vi "HFRR ADV v01.vi"() -> ()   [LabVIEW 2025] (continued)
                      frame #16 {
                        n2627 = Wait (ms)(milliseconds to wait=u32 50) -> ()  [unwired: 1 out]
                      }
                      frame #17 {
                        n2628 = local read "USER ID"() -> (w3679:string)
                        n2629 = Concatenate Strings("Operator ID :" ("Content"), w3679) -> (w3681:string)
                        n2630 = local read "EVENT LOG"() -> (w3683:string)
                        n2631 = call "Event Log.vi"("Content"=w3681, "EVENT LOG"=w3683) -> ("EVENT LOG"=w3682:string)  [unwired: 8 in, 1 out]
                        n2632 = local write "EVENT LOG"(w3682) -> ()
                      }
                      frame #18 {
                        n2633 = Wait (ms)(milliseconds to wait=u32 50) -> ()  [unwired: 1 out]
                      }
                      frame #19 {
                        n2634 = disable-structure shown="Disabled" {
                          frame Disabled {
                            n2635 = local read "EVENT LOG"() -> (w3687:string)
                            n2636 = call "Event Log.vi"("Content"="Test Parameter", "EVENT LOG"=w3687) -> ("EVENT LOG"=w3686:string)  [unwired: 8 in, 1 out]
                            n2637 = local write "EVENT LOG"(w3686) -> ()
                          }
                          frame Enabled {
                          }
                        }
                      }
                      frame #20 {
                        n2638 = Wait (ms)(milliseconds to wait=u32 50) -> ()  [unwired: 1 out]
                      }
                      frame #21 {
                        n2639 = local read "Set Hz"() -> (w3691:dbl)
                        n2640 = Number To Fractional String(number=w3691, precision (6)=i16 2) -> (F-format string=w3690:string)  [unwired: 2 in]
                        n2641 = Concatenate Strings("Set Frequency [Hz] :" ("Content"), w3690) -> (w3693:string)
                        n2642 = local read "EVENT LOG"() -> (w3695:string)
                        n2643 = call "Event Log.vi"("Content"=w3693, "EVENT LOG"=w3695) -> ("EVENT LOG"=w3694:string)  [unwired: 8 in, 1 out]
                        n2644 = local write "EVENT LOG"(w3694) -> ()
                      }
                      frame #22 {
                        n2645 = Wait (ms)(milliseconds to wait=u32 50) -> ()  [unwired: 1 out]
                      }
                      frame #23 {
                        n2646 = local read "NORMAL LOAD"() -> (w3698:dbl)
                        n2647 = Number To Fractional String(number=w3698, precision (6)=i16 2) -> (F-format string=w3699:string)  [unwired: 2 in]
                        n2648 = Concatenate Strings("Applied Load [grams] :" ("Content"), w3699) -> (w3701:string)
                        n2649 = local read "EVENT LOG"() -> (w3703:string)
                        n2650 = call "Event Log.vi"("Content"=w3701, "EVENT LOG"=w3703) -> ("EVENT LOG"=w3702:string)  [unwired: 8 in, 1 out]
                        n2651 = local write "EVENT LOG"(w3702) -> ()
                      }
                      frame #24 {
                        n2652 = Wait (ms)(milliseconds to wait=u32 50) -> ()  [unwired: 1 out]
                      }
                      frame #25 {
                        n2653 = local read "Set Strk"() -> (w3706:dbl)
                        n2654 = Number To Fractional String(number=w3706, precision (6)=i16 2) -> (F-format string=w3707:string)  [unwired: 2 in]
                        n2655 = Concatenate Strings("Set Stroke [mm] :" ("Content"), w3707) -> (w3709:string)
                        n2656 = local read "EVENT LOG"() -> (w3711:string)
                        n2657 = call "Event Log.vi"("Content"=w3709, "EVENT LOG"=w3711) -> ("EVENT LOG"=w3710:string)  [unwired: 8 in, 1 out]
                        n2658 = local write "EVENT LOG"(w3710) -> ()
                      }
                      frame #26 {
                        n2659 = Wait (ms)(milliseconds to wait=u32 50) -> ()  [unwired: 1 out]
                      }
                      frame #27 {
                        n2660 = local read "Set Temp"() -> (w3714:dbl)
                        n2661 = Number To Fractional String(number=w3714, precision (6)=i16 2) -> (F-format string=w3715:string)  [unwired: 2 in]
                        n2662 = Concatenate Strings("Set Temperature [deg C] :" ("Content"), w3715) -> (w3717:string)
                        n2663 = local read "EVENT LOG"() -> (w3719:string)
                        n2664 = call "Event Log.vi"("Content"=w3717, "EVENT LOG"=w3719) -> ("EVENT LOG"=w3718:string)  [unwired: 8 in, 1 out]
                        n2665 = local write "EVENT LOG"(w3718) -> ()
                      }
                      frame #28 {
                        n2666 = Wait (ms)(milliseconds to wait=u32 50) -> ()  [unwired: 1 out]
                      }
                      frame #29 {
                        n2667 = local read "Set Rh"() -> (w3722:dbl)
                        n2668 = Number To Fractional String(number=w3722, precision (6)=i16 2) -> (F-format string=w3723:string)  [unwired: 2 in]
                        n2669 = Concatenate Strings("Set Humidity [%RH] :" ("Content"), w3723) -> (w3725:string)
                        n2670 = local read "EVENT LOG"() -> (w3727:string)
                        n2671 = call "Event Log.vi"("Content"=w3725, "EVENT LOG"=w3727) -> ("EVENT LOG"=w3726:string)  [unwired: 8 in, 1 out]
                        n2672 = local write "EVENT LOG"(w3726) -> ()
                      }
                      frame #30 {
                        n2673 = Wait (ms)(milliseconds to wait=u32 50) -> ()  [unwired: 1 out]
                      }
                      frame #31 {
                        n2674 = local read "test time"() -> (w3730:dbl)
                        n2675 = Number To Fractional String(number=w3730, precision (6)=i16 1) -> (F-format string=w3731:string)  [unwired: 2 in]
                        n2676 = Concatenate Strings("Test Duration [mins] :" ("Content"), w3731) -> (w3733:string)
                        n2677 = local read "EVENT LOG"() -> (w3735:string)
                        n2678 = call "Event Log.vi"("Content"=w3733, "EVENT LOG"=w3735) -> ("EVENT LOG"=w3734:string)  [unwired: 8 in, 1 out]
                        n2679 = local write "EVENT LOG"(w3734) -> ()
                      }
                      frame #32 {
                        w3736 = dbl[] [] ("History Data")
                        w3737 = cluster{"y":dbl, dbl, "y":dbl}[] [] ("History Data")
                        w3738 = FALSE ("Visible")
                        n2680 = property on="Stroke ( mm )" class="WFChart (strict)"("History Data"=w3737) -> ()  [unwired: 2 in, 2 out]
                        n2681 = property on="Temperature ( Deg C )" class="WFChart (strict)"("History Data"=w3736) -> ()  [unwired: 2 in, 2 out]
                        n2682 = property on="Electrical Contact Resistance ( % )" class="WFChart (strict)"("History Data"=w3736) -> ()  [unwired: 2 in, 2 out]
                        n2683 = property on="Coefficient of Friction" class="WFChart (strict)"("History Data"=w3736) -> ()  [unwired: 2 in, 2 out]
                        n2684 = property on="Frictional Force ( N )" class="WFChart (strict)"("History Data"=w3736) -> ()  [unwired: 2 in, 2 out]
                        n2685 = property on="Coefficient of Friction" class="WFChart (strict)"("History Data"=w3736) -> ()  [unwired: 2 in, 2 out]
                        n2686 = property on="Frictional Force ( N )" class="WFChart (strict)"("History Data"=w3736) -> ()  [unwired: 2 in, 2 out]
                        n2687 = property on="Electrical Contact Resistance ( % )" class="WFChart (strict)"("History Data"=w3736) -> ()  [unwired: 2 in, 2 out]
                        n2688 = property on="Stroke ( mm )" class="WFChart (strict)"("History Data"=w3737) -> ()  [unwired: 2 in, 2 out]
                        n2689 = property on="Temperature ( Deg C )" class="WFChart (strict)"("History Data"=w3736) -> ()  [unwired: 2 in, 2 out]
                        n2690 = property on="Service Password Log" class="Str"("Visible"=w3738) -> ()  [unwired: 2 in, 2 out]
                        n2691 = property on="Password 3" class="Clust (strict)"("Visible"=w3738) -> ()  [unwired: 2 in, 2 out]
                      }
                    }
                    n2692 = stacked-sequence {
                      frame #0 {
                        n2693 = local write "Main Dashboard Buttons"(T1."Dashboard" ("Main Dashboard Buttons")) -> ()
                        n2694 = local write "Main Tab"(T4."Acquire" ("Main Tab")) -> ()
                      }
                      frame #1 {
                        n2695 = local write "EVENT LOG"("" ("EVENT LOG")) -> ()
                      }
                      frame #2 {
                        n2696 = Wait (ms)(milliseconds to wait=u32 50) -> ()  [unwired: 1 out]
                      }
                      frame #3 {
                        n2697 = disable-structure shown="Disabled" {
                          frame Disabled {
                            n2698 = local read "EVENT LOG"() -> (w3745:string)
                            n2699 = call "Event Log.vi"("Content"="Test Details", "EVENT LOG"=w3745) -> ("EVENT LOG"=w3744:string)  [unwired: 8 in, 1 out]
                            n2700 = local write "EVENT LOG"(w3744) -> ()
                          }
                          frame Enabled {
                          }
                        }
                      }
                      frame #4 {
                        n2701 = Wait (ms)(milliseconds to wait=u32 50) -> ()  [unwired: 1 out]
                      }
                      frame #5 {
                        n2702 = local read "FILE"() -> (w3747:string)
                        n2703 = Concatenate Strings("File Name :" ("Content"), w3747) -> (w3748:string)
                        n2704 = local read "EVENT LOG"() -> (w3751:string)
                        n2705 = call "Event Log.vi"("Content"=w3748, "EVENT LOG"=w3751) -> ("EVENT LOG"=w3750:string)  [unwired: 8 in, 1 out]
                        n2706 = local write "EVENT LOG"(w3750) -> ()
                      }
                      frame #6 {
                        n2707 = Wait (ms)(milliseconds to wait=u32 50) -> ()  [unwired: 1 out]
                      }
                      frame #7 {
                        n2708 = local read "Batch Ref Num :"() -> (w3753:string)
                        n2709 = Concatenate Strings("Batch Ref No :" ("Content"), w3753) -> (w3754:string)
                        n2710 = local read "EVENT LOG"() -> (w3757:string)
                        n2711 = call "Event Log.vi"("Content"=w3754, "EVENT LOG"=w3757) -> ("EVENT LOG"=w3756:string)  [unwired: 8 in, 1 out]
                        n2712 = local write "EVENT LOG"(w3756) -> ()
                      }
                      frame #8 {
                        n2713 = Wait (ms)(milliseconds to wait=u32 50) -> ()  [unwired: 1 out]
                      }
                      frame #9 {
                        n2714 = local read "tested by"() -> (w3759:string)
                        n2715 = Concatenate Strings("Tested By :" ("Content"), w3759) -> (w3760:string)
                        n2716 = local read "EVENT LOG"() -> (w3763:string)
                        n2717 = call "Event Log.vi"("Content"=w3760, "EVENT LOG"=w3763) -> ("EVENT LOG"=w3762:string)  [unwired: 8 in, 1 out]
                        n2718 = local write "EVENT LOG"(w3762) -> ()
                      }
                      frame #10 {
                        n2719 = Wait (ms)(milliseconds to wait=u32 50) -> ()  [unwired: 1 out]
                      }
                      frame #11 {
                        n2720 = local read "TEST STANDARD"() -> (w3766:T5)
                        n2721 = case shown="\"ASTM D6079\", Default" w3766 {
                          tunnel: ["ASTM D6079" "ISO 12156" "CEC F-096-A-06" "Custom"] -> w3765
                          frame "ASTM D6079", Default {
                          }
                          frame "ISO 12156" {
                          }
                          frame "CEC F-096-A-06" {
                          }
                          frame "Custom" {
                          }
                        }
                        n2722 = Concatenate Strings("Test Standard :" ("Content"), w3765) -> (w3767:string)
                        n2723 = local read "EVENT LOG"() -> (w3770:string)
                        n2724 = call "Event Log.vi"("Content"=w3767, "EVENT LOG"=w3770) -> ("EVENT LOG"=w3769:string)  [unwired: 8 in, 1 out]
                        n2725 = local write "EVENT LOG"(w3769) -> ()
                      }
                      frame #12 {
                        n2726 = Wait (ms)(milliseconds to wait=u32 50) -> ()  [unwired: 1 out]
                      }
                      frame #13 {
                        n2727 = local read "Fuel Discription :"() -> (w3776:string)
                        n2728 = Concatenate Strings("Fuel Description :" ("Content"), w3776) -> (w3777:string)
                        n2729 = local read "EVENT LOG"() -> (w3780:string)
                        n2730 = call "Event Log.vi"("Content"=w3777, "EVENT LOG"=w3780) -> ("EVENT LOG"=w3779:string)  [unwired: 8 in, 1 out]
                        n2731 = local write "EVENT LOG"(w3779) -> ()
                      }
                      frame #14 {
                        n2732 = Wait (ms)(milliseconds to wait=u32 50) -> ()  [unwired: 1 out]
                      }
                      frame #15 {
                        n2733 = local read "Remarks :"() -> (w3782:string)
                        n2734 = Concatenate Strings("Remarks :" ("Content"), w3782) -> (w3783:string)
                        n2735 = local read "EVENT LOG"() -> (w3786:string)
                        n2736 = call "Event Log.vi"("Content"=w3783, "EVENT LOG"=w3786) -> ("EVENT LOG"=w3785:string)  [unwired: 8 in, 1 out]
                        n2737 = local write "EVENT LOG"(w3785) -> ()
                      }
                      frame #16 {
                        n2738 = Wait (ms)(milliseconds to wait=u32 50) -> ()  [unwired: 1 out]
                      }
                      frame #17 {
                        n2739 = local read "USER ID"() -> (w3788:string)
                        n2740 = Concatenate Strings("Operator ID :" ("Content"), w3788) -> (w3790:string)
                        n2741 = local read "EVENT LOG"() -> (w3792:string)
                        n2742 = call "Event Log.vi"("Content"=w3790, "EVENT LOG"=w3792) -> ("EVENT LOG"=w3791:string)  [unwired: 8 in, 1 out]
                        n2743 = local write "EVENT LOG"(w3791) -> ()
                      }
                      frame #18 {
                        n2744 = Wait (ms)(milliseconds to wait=u32 50) -> ()  [unwired: 1 out]
                      }
                      frame #19 {
                        n2745 = disable-structure shown="Disabled" {
                          frame Disabled {
                            n2746 = local read "EVENT LOG"() -> (w3796:string)
                            n2747 = call "Event Log.vi"("Content"="Test Parameter", "EVENT LOG"=w3796) -> ("EVENT LOG"=w3795:string)  [unwired: 8 in, 1 out]
                            n2748 = local write "EVENT LOG"(w3795) -> ()
                          }
                          frame Enabled {
                          }
                        }
                      }
                      frame #20 {
                        n2749 = Wait (ms)(milliseconds to wait=u32 50) -> ()  [unwired: 1 out]
                      }
                      frame #21 {
                        n2750 = local read "Set Hz"() -> (w3800:dbl)
                        n2751 = Number To Fractional String(number=w3800, precision (6)=i16 2) -> (F-format string=w3799:string)  [unwired: 2 in]
                        n2752 = Concatenate Strings("Set Frequency [Hz] :" ("Content"), w3799) -> (w3802:string)
                        n2753 = local read "EVENT LOG"() -> (w3804:string)
                        n2754 = call "Event Log.vi"("Content"=w3802, "EVENT LOG"=w3804) -> ("EVENT LOG"=w3803:string)  [unwired: 8 in, 1 out]
                        n2755 = local write "EVENT LOG"(w3803) -> ()
                      }
                      frame #22 {
                        n2756 = Wait (ms)(milliseconds to wait=u32 50) -> ()  [unwired: 1 out]
                      }
                      frame #23 {
                        n2757 = local read "NORMAL LOAD"() -> (w3807:dbl)
                        n2758 = Number To Fractional String(number=w3807, precision (6)=i16 2) -> (F-format string=w3808:string)  [unwired: 2 in]
                        n2759 = Concatenate Strings("Applied Load [grams] :" ("Content"), w3808) -> (w3810:string)
                        n2760 = local read "EVENT LOG"() -> (w3812:string)
                        n2761 = call "Event Log.vi"("Content"=w3810, "EVENT LOG"=w3812) -> ("EVENT LOG"=w3811:string)  [unwired: 8 in, 1 out]
                        n2762 = local write "EVENT LOG"(w3811) -> ()
                      }
                      frame #24 {
                        n2763 = Wait (ms)(milliseconds to wait=u32 50) -> ()  [unwired: 1 out]
                      }
                      frame #25 {
                        n2764 = local read "Set Strk"() -> (w3815:dbl)
                        n2765 = Number To Fractional String(number=w3815, precision (6)=i16 2) -> (F-format string=w3816:string)  [unwired: 2 in]
                        n2766 = Concatenate Strings("Set Stroke [mm] :" ("Content"), w3816) -> (w3818:string)
                        n2767 = local read "EVENT LOG"() -> (w3820:string)
                        n2768 = call "Event Log.vi"("Content"=w3818, "EVENT LOG"=w3820) -> ("EVENT LOG"=w3819:string)  [unwired: 8 in, 1 out]
                        n2769 = local write "EVENT LOG"(w3819) -> ()
                      }
                      frame #26 {
                        n2770 = Wait (ms)(milliseconds to wait=u32 50) -> ()  [unwired: 1 out]
                      }
                      frame #27 {
                        n2771 = local read "Set Temp"() -> (w3823:dbl)
                        n2772 = Number To Fractional String(number=w3823, precision (6)=i16 2) -> (F-format string=w3824:string)  [unwired: 2 in]
                        n2773 = Concatenate Strings("Set Temperature [deg C] :" ("Content"), w3824) -> (w3826:string)
                        n2774 = local read "EVENT LOG"() -> (w3828:string)
                        n2775 = call "Event Log.vi"("Content"=w3826, "EVENT LOG"=w3828) -> ("EVENT LOG"=w3827:string)  [unwired: 8 in, 1 out]
                        n2776 = local write "EVENT LOG"(w3827) -> ()
                      }
                      frame #28 {
                        n2777 = Wait (ms)(milliseconds to wait=u32 50) -> ()  [unwired: 1 out]
                      }
                      frame #29 {
                        n2778 = local read "Set Rh"() -> (w3831:dbl)
                        n2779 = Number To Fractional String(number=w3831, precision (6)=i16 2) -> (F-format string=w3832:string)  [unwired: 2 in]
                        n2780 = Concatenate Strings("Set Humidity [%RH] :" ("Content"), w3832) -> (w3834:string)
                        n2781 = local read "EVENT LOG"() -> (w3836:string)
                        n2782 = call "Event Log.vi"("Content"=w3834, "EVENT LOG"=w3836) -> ("EVENT LOG"=w3835:string)  [unwired: 8 in, 1 out]
                        n2783 = local write "EVENT LOG"(w3835) -> ()
                      }
                      frame #30 {
                        n2784 = Wait (ms)(milliseconds to wait=u32 50) -> ()  [unwired: 1 out]
                      }
                      frame #31 {
                        n2785 = local read "test time"() -> (w3839:dbl)
                        n2786 = Number To Fractional String(number=w3839, precision (6)=i16 1) -> (F-format string=w3840:string)  [unwired: 2 in]
                        n2787 = Concatenate Strings("Test Duration [mins] :" ("Content"), w3840) -> (w3842:string)
                        n2788 = local read "EVENT LOG"() -> (w3844:string)
                        n2789 = call "Event Log.vi"("Content"=w3842, "EVENT LOG"=w3844) -> ("EVENT LOG"=w3843:string)  [unwired: 8 in, 1 out]
                        n2790 = local write "EVENT LOG"(w3843) -> ()
                      }
                      frame #32 {
                        w3845 = dbl[] [] ("History Data")
                        w3846 = cluster{"y":dbl, dbl, "y":dbl}[] [] ("History Data")
                        w3847 = FALSE ("Visible")
                        n2791 = property on="Stroke ( mm )" class="WFChart (strict)"("History Data"=w3846) -> ()  [unwired: 2 in, 2 out]
                        n2792 = property on="Temperature ( Deg C )" class="WFChart (strict)"("History Data"=w3845) -> ()  [unwired: 2 in, 2 out]
                        n2793 = property on="Electrical Contact Resistance ( % )" class="WFChart (strict)"("History Data"=w3845) -> ()  [unwired: 2 in, 2 out]
                        n2794 = property on="Coefficient of Friction" class="WFChart (strict)"("History Data"=w3845) -> ()  [unwired: 2 in, 2 out]
                        n2795 = property on="Frictional Force ( N )" class="WFChart (strict)"("History Data"=w3845) -> ()  [unwired: 2 in, 2 out]
                        n2796 = property on="Coefficient of Friction" class="WFChart (strict)"("History Data"=w3845) -> ()  [unwired: 2 in, 2 out]
                        n2797 = property on="Frictional Force ( N )" class="WFChart (strict)"("History Data"=w3845) -> ()  [unwired: 2 in, 2 out]
                        n2798 = property on="Electrical Contact Resistance ( % )" class="WFChart (strict)"("History Data"=w3845) -> ()  [unwired: 2 in, 2 out]
                        n2799 = property on="Stroke ( mm )" class="WFChart (strict)"("History Data"=w3846) -> ()  [unwired: 2 in, 2 out]
                        n2800 = property on="Temperature ( Deg C )" class="WFChart (strict)"("History Data"=w3845) -> ()  [unwired: 2 in, 2 out]
                        n2801 = property on="Service Password Log" class="Str"("Visible"=w3847) -> ()  [unwired: 2 in, 2 out]
                        n2802 = property on="Password 3" class="Clust (strict)"("Visible"=w3847) -> ()  [unwired: 2 in, 2 out]
                      }
                    }
                    "TEST FILE NAM,E SAVED" <- TRUE ("TEST FILE NAM,E SAVED")
                  }
                }
              }
            }
          }
        }
        n2803 = case shown="Default" w3110 {
          tunnel: w3112 -> [_ w3215]
          frame Default {
            n2804 = property on="DEMO" class="Bool (strict)"() -> ("Value"=w3212:bool)  [unwired: 2 in, 2 out]
            n2805 = case shown="False" w3212 {
              frame False {
                w3214 = 0.0 ("output")
                n2806 = local write "PID-out"(w3214) -> ()
                n2807 = local write "Frequency ( Hz )"(w3214) -> ()
              }
              frame True {
              }
            }
            n2808 = local write "STROKE Initialize"(TRUE ("STROKE Initialize")) -> ()
          }
          frame "Acquire" {
            n2809 = stacked-sequence {
              frame #0 {
                n2810 = property on="DEMO" class="Bool (strict)"() -> ("Value"=w3217:bool)  [unwired: 2 in, 2 out]
                n2811 = case shown="False" w3217 {
                  frame False {
                    n2812 = local read "Auto Start Test"() -> (w3218:bool)
                    n2813 = case shown="True" w3218 {
                      tunnel: "RUN" -> [w3239 w3242]
                      tunnel: [w3239 w3241] -> w3219
                      frame False {
                      }
                      frame True {
                        n2814 = local read "Auto Start Temp"() -> (w3240:bool)
                        n2815 = Or(x=w3242, y=w3240) -> (x .or. y?=w3241:bool)
                      }
                    }
                    n2816 = local read "clk"() -> (w3238:dbl)
                    n2817 = local read "Save"() -> (w3234:bool)
                    n2818 = Equal?(x=w3238, y=0.0) -> (x = y?=w3235:bool)
                    n2819 = And(x=w3235, y=w3234) -> (x .and. y?=w3236:bool)
                    n2820 = Not(x="Engage") -> (.not. x?=w3225:bool)
                    n2821 = case shown="False" w3219 {
                      tunnel: [0.0 w3266] -> w3221
                      frame False {
                        (unwired) TRUE ("Visible")
                        n2822 = local read "Auto Start Test"() -> (w3246:bool)
                        n2823 = local write "Start Time"(TRUE ("Start Time")) -> ()
                        n2824 = property on="Stroke 2" class="DigNum (strict)"("Visible"=FALSE) -> ()  [unwired: 2 in, 2 out]
                        n2825 = case shown="False" w3246 {
                          frame False {
                            n2826 = property on="Heater Button" class="Bool (strict)"("DisabledEnum"=T20."Enabled" ("Disabled")) -> ()  [unwired: 2 in, 2 out]
                            n2827 = property on="Humidity" class="Bool (strict)"("DisabledEnum"=T20."Enabled" ("Disabled")) -> ()  [unwired: 2 in, 2 out]
                          }
                          frame True {
                          }
                        }
                        n2828 = case shown="False" "TestCompFlg" {
                          frame False {
                            n2829 = local read "StartFlg"() -> (w3254:bool)
                            n2830 = case shown="True" w3254 {
                              frame False {
                              }
                              frame True {
                                n2831 = stacked-sequence {
                                frame #0 {
                                n2832 = local read "EVENT LOG"() -> (w3258:string)
                                n2833 = call "Event Log.vi"("Content"="Test was interrupted", "EVENT LOG"=w3258) -> ("EVENT LOG"=w3259:string)  [unwired: 8 in, 1 out]
                                n2834 = local write "EVENT LOG"(w3259) -> ()
                                n2835 = property on="RUN" class="Bool (strict)"("Visible"=TRUE) -> ()  [unwired: 2 in, 2 out]
                                n2836 = property on="Auto Start Test" class="Bool (strict)"("Visible"=TRUE) -> ()  [unwired: 2 in, 2 out]
                                }
                                frame #1 {
                                w3262 = FALSE ("StartFlg")
                                n2837 = property on="Heater Button" class="Bool (strict)"("Val(Sgnl)"=FALSE ("Value (Signaling)")) -> ()  [unwired: 2 in, 2 out]
                                n2838 = local write "Heater Button"(w3262) -> ()
                                n2839 = local write "StartFlg"(w3262) -> ()
                                n2840 = local write "Humidity"(w3262) -> ()
                                n2841 = local write "Humidity 2"(TRUE ("Humidity")) -> ()
                                }
                                frame #2 {
                                n2842 = local write "Due Write"("VC;0" ("Command")) -> ()
                                }
                                frame #3 {
                                n2843 = Wait (ms)(milliseconds to wait=u32 1500) -> ()  [unwired: 1 out]
                                }
                                frame #4 {
                                n2844 = local write "Due Write"("HE;0" ("Command")) -> ()
                                }
                                }
                              }
                            }
                          }
                          frame True {
                          }
                        }
                        n2845 = local write "String 14"("Test will autostart once parameters reach the set value." ("String 14")) -> ()
                      }
                      frame True {
                        (unwired) FALSE ("Visible")
                        n2846 = property on="Stroke 2" class="DigNum (strict)"("Visible"=TRUE) -> ()  [unwired: 2 in, 2 out]
                        n2847 = property on="STOP 2" class="Bool (strict)"("Disabled"=u8 2) -> ()  [unwired: 2 in, 2 out]
                        n2848 = local write "String 14"(" Running....." ("String 14")) -> ()
                        n2849 = property on="Heater Button" class="Bool (strict)"("DisabledEnum"=T20."Disabled and Grayed Out" ("Disabled")) -> ()  [unwired: 2 in, 2 out]
                        n2850 = property on="Humidity" class="Bool (strict)"("DisabledEnum"=T20."Disabled and Grayed Out" ("Disabled")) -> ()  [unwired: 2 in, 2 out]
                        n2851 = case shown="True" "Start Time" {
                          selector: "Start Time" -> [_ w3285]
                          frame False {
                          }
                          frame True {
                            n2852 = Not(x=w3285) -> (.not. x?=w3284:bool)
                            n2853 = local write "Start Time"(w3284) -> ()
                            n2854 = local read "EVENT LOG"() -> (w3286:string)
                            n2855 = call "Event Log.vi"("Content"="Test in progress", "EVENT LOG"=w3286) -> ("EVENT LOG"=w3288:string)  [unwired: 8 in, 1 out]
                            n2856 = local write "EVENT LOG"(w3288) -> ()
                          }
                        }
                        n2857 = disable-structure shown="Enabled" {
                          disable-tunnel: [w3277 w3283] -> w3266
                          frame Disabled {
                            n2858 = local read "Set Hz"() -> (w3280:dbl)
                            n2859 = call <vilib>:"Uniform White Noise Waveform.vi"() -> ("signal out"=w3279:waveform(dbl))  [unwired: 10 in, 1 out]
                            n2860 = Random Number (0-1)() -> (number: 0 to 1=w3276:dbl)
                            n2861 = Add(x=w3280, y=w3279) -> (x+y=w3278:waveform(dbl))
                            n2862 = Multiply(x=ext 0.01 ("y"), y=w3276) -> (x*y=w3274:ext)
                            n2863 = Multiply(x=w3278, y=w3274) -> (x*y=w3277:waveform(ext))
                          }
                          frame Enabled {
                            n2864 = call-poly <vilib>:"Random Number (Range).vi"("lower bound (0)"=49.89, "upper bound (100)"=50.8) -> ("number"=w3283:dbl)  [unwired: 9 in]
                          }
                        }
                        "StartFlg" <- TRUE ("StartFlg")
                      }
                    }
                    n2865 = case shown="True" w3236 {
                      frame False {
                      }
                      frame True {
                        n2866 = local write "clk"(10.0 ("clk")) -> ()
                        n2867 = Get Date/Time In Seconds() -> (seconds since 1Jan1904=w3291:timestamp)
                        n2868 = To Double Precision Float(number=w3291) -> (double precision float=w3289:dbl)
                        n2869 = local write "acq timer"(w3289) -> ()
                        n2870 = local write "act save time"(w3289) -> ()
                      }
                    }
                    n2871 = call "Elapsed Time"("Time Target (s)"="Countdown", "Reset"=w3225) -> ("Elapsed Time (s)"=w3230:dbl, "Time has Elapsed"=w3228:bool)  [unwired: 10 in, 6 out]
                    "Countdown 2" <- w3230
                    n2872 = Subtract(x=w3230, y=2.0) -> (x-y=w3233:dbl)
                    n2873 = Less?(x=w3233, y="Countdown") -> (x < y?=w3231:bool)
                    n2874 = And(x=w3231, y=w3228) -> (x .and. y?=w3227:bool)
                    n2875 = case shown="True" w3227 {
                      frame False {
                      }
                      frame True {
                        (unwired) dbl[] [] ("History Data")
                        n2876 = local write "Engage"(FALSE ("Engage")) -> ()
                        n2877 = local write "RUN"(TRUE ("RUN")) -> ()
                        n2878 = local read "Humidity ( %RH )"() -> (→"Rh Before":dbl)
                      }
                    }
                    n2879 = local read "Test \nStatus"() -> (w3223:bool)
                    n2880 = Select(t=w3221, s=w3223, f=0.0) -> (s? t:f=w3222:dbl)
                    n2881 = local write "Frequency ( Hz )"(w3222) -> ()
                  }
                  frame True {
                  }
                }
              }
              frame #1 {
                # "HC;1/0\nST;VALUE"
                # "Elapsed time\ncof\nstroke\nAir temp\nTemp\nHumidity"
                # "acq timer\n\nact save time"
                # "convert to microseconds"
                n2882 = property on="DEMO" class="Bool (strict)"() -> ("Value"=w3292:bool)  [unwired: 2 in, 2 out]
                n2883 = case shown="True" w3292 {
                  tunnel: [w3310 FALSE] -> w3297
                  tunnel: [w3309 0.0] -> w3296
                  frame False {
                    w3317 = 1000000.0 ("x")
                    n2884 = local read "Rate"() -> (w3313:dbl)
                    n2885 = Divide(x=w3317, y=w3313) -> (x/y=w3318:dbl)
                    n2886 = Get Date/Time In Seconds() -> (seconds since 1Jan1904=w3320:timestamp)
                    n2887 = local read "Samplingtime 2"() -> (w3301:dbl)
                    n2888 = local read "act save time"() -> (w3315:dbl)
                    n2889 = Divide(x=w3318, y=w3317) -> (x/y=w3316:dbl)
                    n2890 = To Double Precision Float(number=w3320) -> (double precision float=w3309:dbl)
                    n2891 = Add(x=w3315, y=w3301) -> (x+y=w3314:dbl)
                    n2892 = local read "acq timer"() -> (w3319:dbl)
                    n2893 = local read "COUNT"() -> (w3302:i32)
                    n2894 = Greater Or Equal?(x=w3309, y=w3314) -> (x >= y?=w3300:bool)
                    n2895 = Multiply(x=w3316, y=w3302) -> (x*y=w3308:dbl)
                    n2896 = Subtract(x=w3309, y=w3319) -> (x-y=w3311:dbl)
                    n2897 = local read "Save"() -> (w3312:bool)
                    n2898 = Add(x=w3311, y=w3308) -> (x+y=w3298:dbl)
                    "Elapsed time 3" <- w3298
                    n2899 = And(x=w3300, y=w3312) -> (x .and. y?=w3310:bool)
                    n2900 = Divide(x=w3298, y=60.0) -> (x/y=w3306:dbl)
                    n2901 = local read "Test \nStatus"() -> (w3299:bool)
                    n2902 = local read "clk"() -> (w3303:dbl)
                    n2903 = Equal?(x=w3303, y=10.0) -> (x = y?=w3305:bool)
                    n2904 = case shown="True" w3299 {
                      tunnel: w3306 -> [_ w3329]
                      tunnel: w3311 -> [_ w3339]
                      tunnel: [0.0 w3335] -> _
                      tunnel: w3305 -> [_ w3334]
                      tunnel: [0.0 w3333] -> _
                      tunnel: w3298 -> [_ w3333]
                      tunnel: w3309 -> [w3322 _]
                      frame False {
                        n2905 = local write "acq timer"(w3322) -> ()
                        n2906 = local write "Test Duration Status"(0.0 ("Test Duration Status")) -> ()
                      }
                      frame True {
                        n2907 = local write "Elapsed time"(w3329) -> ()
                        n2908 = local read "Set Hz"() -> (w3336:dbl)
                        n2909 = local read "test time"() -> (w3328:dbl)
                        n2910 = Multiply(x=w3339, y=w3336) -> (x*y=w3338:dbl)
                        n2911 = Greater?(x=w3329, y=w3328) -> (0:w3337:bool)
                        n2912 = Subtract(x=w3328, y=w3329) -> (x-y=w3327:dbl)
                        n2913 = case shown="False" w3334 {
                          tunnel: w3338 -> [w3340 _]
                          tunnel: [w3340 1.0] -> w3335
                          frame False {
                            n2914 = local write "Cycles elapsed"(w3340) -> ()
                          }
                          frame True {
                          }
                        }
                        n2915 = Multiply(x=w3327, y=60.0) -> (x*y=w3326:dbl)
                        n2916 = local write "Time Remaining"(w3326) -> ()
                        n2917 = local write "Remaining Time"(w3326) -> ()
                        n2918 = case shown="True" w3337 {
                          frame False {
                          }
                          frame True {
                            n2919 = stacked-sequence {
                              frame #0 {
                                w3345 = T20."Enabled" ("Disabled")
                                w3344 = FALSE ("TEST FILE NAM,E SAVED")
                                w3346 = "" ("FILE")
                                w3347 = TRUE ("Visible")
                                n2920 = local write "Humidity"(FALSE ("Humidity")) -> ()
                                n2921 = local write "RUN"(FALSE ("OK Button 2")) -> ()
                                n2922 = local write "Heater Button"(FALSE ("Heater Button")) -> ()
                                n2923 = local write "Auto Start Test"(FALSE ("Auto Start Test")) -> ()
                                n2924 = local write "TestCompFlg"(TRUE ("StpFlg")) -> ()
                                n2925 = local read "Humidity ( %RH )"() -> (→"Rh After":dbl)
                                n2926 = property on="STOP 2" class="Bool (strict)"("Disabled"=u8 0) -> ()  [unwired: 2 in, 2 out]
                                n2927 = local read "EVENT LOG"() -> (w3352:string)
                                n2928 = call "Event Log.vi"("Content"="Test Completed", "EVENT LOG"=w3352) -> ("EVENT LOG"=w3351:string)  [unwired: 8 in, 1 out]
                                n2929 = property on="RUN" class="Bool (strict)"("Visible"=w3347) -> ()  [unwired: 2 in, 2 out]
                                n2930 = property on="Auto Start Test" class="Bool (strict)"("Visible"=w3347) -> ()  [unwired: 2 in, 2 out]
                                n2931 = local write "Batch Ref Num :"(w3346) -> ()
                                n2932 = local write "FILE"(w3346) -> ()
                                n2933 = local write "EVENT LOG"(w3351) -> ()
                                n2934 = local write "TEST FILE NAM,E SAVED"(w3344) -> ()
                                n2935 = local write "Fuel Discription :"(w3346) -> ()
                                n2936 = local write "START TEMP"(w3344) -> ()
                                n2937 = local write "Remarks :"(w3346) -> ()
                                n2938 = local write "Main Dashboard Buttons"(T1."Imaging" ("Main Dashboard Buttons")) -> ()
                                n2939 = local write "Main Tab"(T4."Adv Scar" ("Main Tab")) -> ()
                                n2940 = property on="FRICVALZ 2" class="Bool (strict)"("DisabledEnum"=w3345) -> ()  [unwired: 2 in, 2 out]
                                n2941 = property on="FRICVALZ 3" class="Bool (strict)"("DisabledEnum"=w3345) -> ()  [unwired: 2 in, 2 out]
                                n2942 = property on="FRICVALZ 4" class="Bool (strict)"("DisabledEnum"=w3345) -> ()  [unwired: 2 in, 2 out]
                              }
                              frame #1 {
                                n2943 = Wait (ms)(milliseconds to wait=u32 2000) -> ()  [unwired: 1 out]
                              }
                              frame #2 {
                                n2944 = local write "Due Write"("VC;0") -> ()
                              }
                              frame #3 {
                                n2945 = Wait (ms)(milliseconds to wait=u32 2000) -> ()  [unwired: 1 out]
                              }
                              frame #4 {
                                n2946 = local write "Due Write"("VC;0") -> ()
                              }
                              frame #5 {
                                n2947 = Wait (ms)(milliseconds to wait=u32 2000) -> ()  [unwired: 1 out]
                              }
                              frame #6 {
                                n2948 = local write "Due Write"("ST;0") -> ()
                              }
                              frame #7 {
                                n2949 = local write "measured_stroke"(0.0 ("measured_stroke")) -> ()
                                n2950 = Wait (ms)(milliseconds to wait=u32 1500) -> ()  [unwired: 1 out]
                              }
                              frame #8 {
                                n2951 = local write "Due Write"("HE;0") -> ()
                                n2952 = local write "Humidity 2"(TRUE ("Humidity")) -> ()
                              }
                            }
                          }
                        }
                        n2953 = Divide(x=w3329, y=w3328) -> (x/y=w3332:dbl)
                        n2954 = Multiply(x=w3332, y=100.0) -> (x*y=w3330:dbl)
                        n2955 = local write "Test Duration Status"(w3330) -> ()
                      }
                    }
                  }
                  frame True {
                  }
                }
                n2956 = local read "COUNT"() -> (w3294:i32)
                n2957 = Greater Or Equal?(x=w3294, y=250) -> (x >= y?=w3293:bool)
                n2958 = case shown="True" w3293 {
                  frame False {
                    n2959 = local read "COUNT"() -> (w3370:i32)
                    n2960 = Increment(x=w3370) -> (x+1=w3371:i32)
                    n2961 = local write "COUNT"(w3371) -> ()
                  }
                  frame True {
                    n2962 = local write "COUNT"(0 ("COUNT")) -> ()
                  }
                }
                n2963 = case shown="True" w3297 {
                  tunnel: w3296 -> [_ w3438]
                  tunnel: [FALSE ("Boolean 2") TRUE ("Boolean 2")] -> _
                  frame False {
                  }
                  frame True {
                    w3392 = ";" ("Substring")
                    # "Pid out/\nFreq response value"
                    n2964 = local write "act save time"(w3438) -> ()
                    n2965 = local read "FILE"() -> (w3386:string)
                    n2966 = call "file check.vi"("file name in"=w3386) -> ("error out"=w3389:errorcluster, "file name out"=w3384:string)  [unwired: 9 in]
                    n2967 = local read "LVDT STROKE"() -> (w3381:dbl)
                    n2968 = local read "Add up Stroke"() -> (w3379:dbl)
                    n2969 = call "FILE PATH CREATION.vi"("error in"=w3389, "FILE NAME :"=w3384) -> ("FILE OUT"=w3387:path)  [unwired: 8 in, 1 out]
                    n2970 = local read "STROKE Initialize"() -> (w3374:bool)
                    n2971 = Concatenate Strings(w3384, ".dgf" ("Substring")) -> (w3388:string)
                    n2972 = Subtract(x=w3381, y=w3379) -> (x-y=w3380:dbl)
                    n2973 = Absolute Value(x=w3380) -> (abs(x)=w3377:dbl)
                    n2974 = local read "FF 2"() -> (→"Frictional Force ( N )" →"Frictional Force ( N )":dbl)
                    n2975 = Build Path(base path=w3387, name or relative path=w3388) -> (appended path=w3383:path)
                    n2976 = flat-sequence {
                      tunnel: w3377 -> [w3443]
                      tunnel: [w3442] -> w3375
                      tunnel: w3374 -> [w3440]
                      tunnel: [w3445] -> w3376
                      tunnel: w3375 -> [w3445]
                      frame #0 {
                        n2977 = call <vilib>:"Mean PtByPt.vi"("x"=w3443, "sample length"="STROKE FILTER", "initialize"=w3440) -> ("mean"=w3442:dbl)  [unwired: 1 in, 1 out]
                      }
                      frame #1 {
                        "STROKE Initialize" <- FALSE ("STROKE Initialize")
                      }
                    }
                    n2978 = local read "COF 2"() -> (w3397:dbl)
                    "Coefficient of Friction" <- w3397
                    "COF 4" <- w3397
                    "Coefficient of Friction" <- w3397
                    n2979 = local read "TEMP"() -> (w3400:dbl)
                    "Temperature ( Deg C )" <- w3400
                    n2980 = local read "Humidity ( %RH )"() -> (w3399:dbl)
                    n2981 = local read "Frequency ( Hz )"() -> (w3406:dbl)
                    n2982 = local read "LVDT STROKE DISPLAY"() -> (w3378:dbl)
                    n2983 = local read "Elapsed time"() -> (w3431:dbl)
                    n2984 = local read "AIR TEMP"() -> (w3404:dbl)
                    n2985 = local read "PID-out"() -> (w3409:dbl)
                    n2986 = local write "Temperature ( Deg C )"(w3400) -> ()
                    n2987 = Number To Fractional String(number=w3378, width (-)=i16 9 ("precision (6)"), precision (6)=i16 6) -> (F-format string=w3424:string)  [unwired: 1 in]
                    n2988 = Number To Fractional String(number=w3404, width (-)=i16 9 ("precision (6)"), precision (6)=i16 3) -> (F-format string=w3423:string)  [unwired: 1 in]
                    n2989 = Number To Fractional String(number=w3400, width (-)=i16 9 ("precision (6)"), precision (6)=i16 3) -> (F-format string=w3420:string)  [unwired: 1 in]
                    n2990 = Number To Fractional String(number=w3399, width (-)=i16 9 ("precision (6)"), precision (6)=i16 3) -> (F-format string=w3417:string)  [unwired: 1 in]
                    n2991 = Number To Fractional String(number=0.0, width (-)=i16 9 ("precision (6)"), precision (6)=i16 3) -> (F-format string=w3414:string)  [unwired: 1 in]
                    n2992 = Number To Fractional String(number=w3409, width (-)=i16 9 ("precision (6)"), precision (6)=i16 3) -> (F-format string=w3410:string)  [unwired: 1 in]
                    n2993 = Number To Fractional String(number=w3406, width (-)=i16 9 ("precision (6)"), precision (6)=i16 3) -> (F-format string=w3405:string)  [unwired: 1 in]
                    n2994 = Number To Fractional String(number=w3397, width (-)=i16 9 ("precision (6)"), precision (6)=i16 6) -> (F-format string=w3432:string)  [unwired: 1 in]
                    n2995 = Number To Fractional String(number=w3431, width (-)=i16 14 ("precision (6)"), precision (6)=i16 3) -> (F-format string=w3433:string)  [unwired: 1 in]
                    n2996 = Bundle("y"=1.02, "LVDT STROKE DISPLAY"=w3378, "y"=0.98) -> (w3398:T31)  [unwired: 1 in]
                    n2997 = Number To Fractional String(number="Ambient Humidity :", width (-)=i16 9 ("precision (6)"), precision (6)=i16 6) -> (F-format string=w3390:string)  [unwired: 1 in]
                    n2998 = local read "RUN"() -> (w3396:bool)
                    n2999 = case shown="True" w3396 {
                      tunnel: w3398 -> [_ w3449]
                      tunnel: w3378 -> [_ w3448]
                      tunnel: w3378 -> [_ w3446]
                      tunnel: w3378 -> [_ w3447]
                      frame False {
                      }
                      frame True {
                        "Stroke ( mm )" <- w3449
                        "Stroke ( mm )" <- w3449
                        "Stroke 4" <- w3448
                        "Stroke 3" <- w3446
                        "Stroke 2" <- w3447
                        "measured_stroke" <- w3446
                      }
                    }
                    n3000 = Concatenate Strings(w3433, w3392, w3432, w3392, w3424, w3392, w3423, w3392, w3420, w3392, w3417, w3392, w3414, w3392, w3410, w3392, w3405, w3392, w3390, "\r") -> (w3430:string)
                    n3001 = call <vilib>:"Write Characters To File.vi"("append to file? (new file:F)"=TRUE, "character string"=w3430, "file path (dialog if empty)"=w3383) -> ()  [unwired: 2 in, 1 out]
                    "refresh flag" <- TRUE ("refresh flag")
                    "LVDT STROKE Actual" <- w3376
                  }
                }
              }
              frame #2 {
                n3002 = case shown="True" "Heater Button" {
                  tunnel: [0.0 ("output") w3472] -> w3450
                  frame False {
                    w3453 = TRUE ("tmpchk")
                    n3003 = local read "TEMP"() -> (w3454:dbl)
                    n3004 = local write "Temp ini"(w3454) -> ()
                    n3005 = local write "Reset 4"(w3453) -> ()
                    n3006 = local write "tmpchk"(w3453) -> ()
                    n3007 = local write "reinit"(TRUE ("reinit")) -> ()
                    n3008 = local write "manual temp log"(TRUE ("manual temp log")) -> ()
                  }
                  frame True {
                    # "Logic to turn off\nthe heater when \ntemp is not rising.\nTime - 60 sec\nDelta t- 5°c"
                    n3009 = local read "Temp ini"() -> (w3461:dbl)
                    n3010 = local read "Auto Start Test"() -> (w3457:bool)
                    n3011 = Less?(x=w3461, y=53.0) -> (x < y?=w3459:bool)
                    n3012 = case shown="False" w3457 {
                      frame False {
                        n3013 = local read "Set Temp"() -> (w3481:dbl)
                        n3014 = local read "TEMP"() -> (w3480:dbl)
                        n3015 = Subtract(x=w3481, y=w3480) -> (x-y=w3479:dbl)
                        n3016 = Absolute Value(x=w3479) -> (abs(x)=w3478:dbl)
                        n3017 = Less?(x=w3478, y=0.5) -> (x < y?=w3476:bool)
                        n3018 = case shown="True" w3476 {
                          tunnel: "manual temp log" -> [_ w3482]
                          frame False {
                          }
                          frame True {
                            n3019 = case shown="True" w3482 {
                              selector: w3482 -> [_ w3483]
                              frame False {
                              }
                              frame True {
                                # "#Event log"
                                n3020 = Not(x=w3483) -> (.not. x?=w3484:bool)
                                n3021 = local write "manual temp log"(w3484) -> ()
                                n3022 = local read "EVENT LOG"() -> (w3487:string)
                                n3023 = call "Event Log.vi"("Content"="Target Temperature reached", "EVENT LOG"=w3487) -> ("EVENT LOG"=w3486:string)  [unwired: 8 in, 1 out]
                                n3024 = local write "EVENT LOG"(w3486) -> ()
                              }
                            }
                          }
                        }
                      }
                      frame True {
                        n3025 = local write "manual temp log"(TRUE ("manual temp log")) -> ()
                      }
                    }
                    n3026 = And(x="tmpchk", y=w3459) -> (x .and. y?=w3462:bool)
                    n3027 = case shown="True" w3462 {
                      frame False {
                      }
                      frame True {
                        n3028 = call "Elapsed Time8"("Time Target (s)"=300.0, "Reset"="Reset 4") -> ("Time has Elapsed"=w3489:bool)  [unwired: 10 in, 7 out]
                        n3029 = flat-sequence {
                          tunnel: w3489 -> [_]
                          frame #0 {
                            n3030 = local write "Reset 4"(FALSE ("Reset 4")) -> ()
                          }
                        }
                        n3031 = case shown="True" w3489 {
                          frame False {
                          }
                          frame True {
                            n3032 = local read "Temp ini"() -> (w3496:dbl)
                            n3033 = Add(x=w3496, y=5.0) -> (x+y=w3494:dbl)
                            n3034 = local read "TEMP"() -> (w3497:dbl)
                            n3035 = Greater?(x=w3497, y=w3494) -> (0:w3495:bool)
                            n3036 = case shown="False" w3495 {
                              frame False {
                                n3037 = local write "Heater Button"(FALSE ("Heater Button")) -> ()
                              }
                              frame True {
                                n3038 = local write "tmpchk"(FALSE ("tmpchk")) -> ()
                              }
                            }
                          }
                        }
                      }
                    }
                    n3039 = local read "Set Temp"() -> (w3470:dbl)
                    n3040 = local read "TEMP"() -> (w3464:dbl)
                    n3041 = call-poly <vilib>:"PID.vi"("reinitialize? (F)"="reinit", "dt (s)"=-1.0, "process variable"=w3464, "setpoint"=w3470) -> ("output"=w3467:dbl)  [unwired: 6 in, 1 out]
                    n3042 = Subtract(x=w3470, y=w3464) -> (x-y=w3471:dbl)
                    n3043 = Add(x=w3470, y=0.5) -> (x+y=w3468:dbl)
                    n3044 = Greater Or Equal?(x=w3464, y=w3468) -> ()  [unwired: 1 out]
                    n3045 = Select(t=0.0, s=FALSE, f=w3467) -> (s? t:f=w3466:dbl)
                    "PID output" <- w3466
                    n3046 = flat-sequence {
                      tunnel: w3466 -> [w3500]
                      tunnel: [w3500] -> w3472
                      frame #0 {
                        n3047 = local write "reinit"(FALSE ("reinit")) -> ()
                      }
                    }
                    n3048 = Bundle(w3471, "output"=w3466, "TEMP"=w3464) -> ()  [unwired: 1 in, 1 out]
                  }
                }
                "PID-out" <- w3450
              }
              frame #3 {
                n3049 = local read "TEMP"() -> (w3502:dbl)
                n3050 = Greater Or Equal?(x=w3502, y="Set Temp 2") -> (x >= y?=w3507:bool)
                n3051 = case shown="True" w3507 {
                  tunnel: [FALSE TRUE] -> w3505
                  frame False {
                  }
                  frame True {
                  }
                }
                "Status 13" <- w3505
                n3052 = And(x=w3505, y="trip1 8") -> (x .and. y?=w3504:bool)
                n3053 = case shown="True" w3504 {
                  frame False {
                    n3054 = local write "Heater Trip Temp"(TRUE ("Heater Trip Temp")) -> ()
                  }
                  frame True {
                    w3510 = FALSE ("OK Button 2")
                    n3055 = case shown="True" "Heater Trip Temp" {
                      selector: "Heater Trip Temp" -> [_ w3512]
                      frame False {
                      }
                      frame True {
                        n3056 = Not(x=w3512) -> (.not. x?=w3511:bool)
                        n3057 = local read "EVENT LOG"() -> (w3515:string)
                        n3058 = local write "Heater Trip Temp"(w3511) -> ()
                        n3059 = call "Event Log.vi"("Content"="Heater Trip", "EVENT LOG"=w3515) -> ("EVENT LOG"=w3514:string)  [unwired: 8 in, 1 out]
                        n3060 = local write "EVENT LOG"(w3514) -> ()
                      }
                    }
                    n3061 = local write "RUN"(w3510) -> ()
                    n3062 = property on="Auto Start Test" class="Bool (strict)"("Value"=w3510) -> ()  [unwired: 2 in, 2 out]
                    n3063 = local write "Heater Button"(w3510) -> ()
                  }
                }
              }
            }
            n3064 = case shown="False" w3215 {
              frame False {
                n3065 = disable-structure shown="Disabled" {
                  frame Disabled {
                    n3066 = stacked-sequence {
                      frame #0 {
                        n3067 = local write "RUN"(FALSE ("OK Button 2")) -> ()
                      }
                      frame #1 {
                      }
                    }
                  }
                  frame Enabled {
                  }
                }
              }
              frame True {
              }
            }
          }
        }
        n3068 = local write "Test \nStatus"(w3116) -> ()
        n3069 = local write "Save"(w3116) -> ()
        n3070 = case shown="True" w3113 {
          frame False {
            n3071 = local read "Rt 3"() -> (w3184:bool)
